vi "Test - Baum Welch algorithm.vi"() -> ()   [LabVIEW 2014, in "HMM.lvlib"]
uses:
  HMM.lvlib
panel:
  out "Estimated HMM 2":T1
  out "#iterations":i32
  out "Probability":dbl[](graph)
  out "Estimated HMM":T1
  out "Observed states":i32[](graph)
  in  "Length of observation":i32
  in  "#iterations":i32=100
  in  "Test HMM":T1
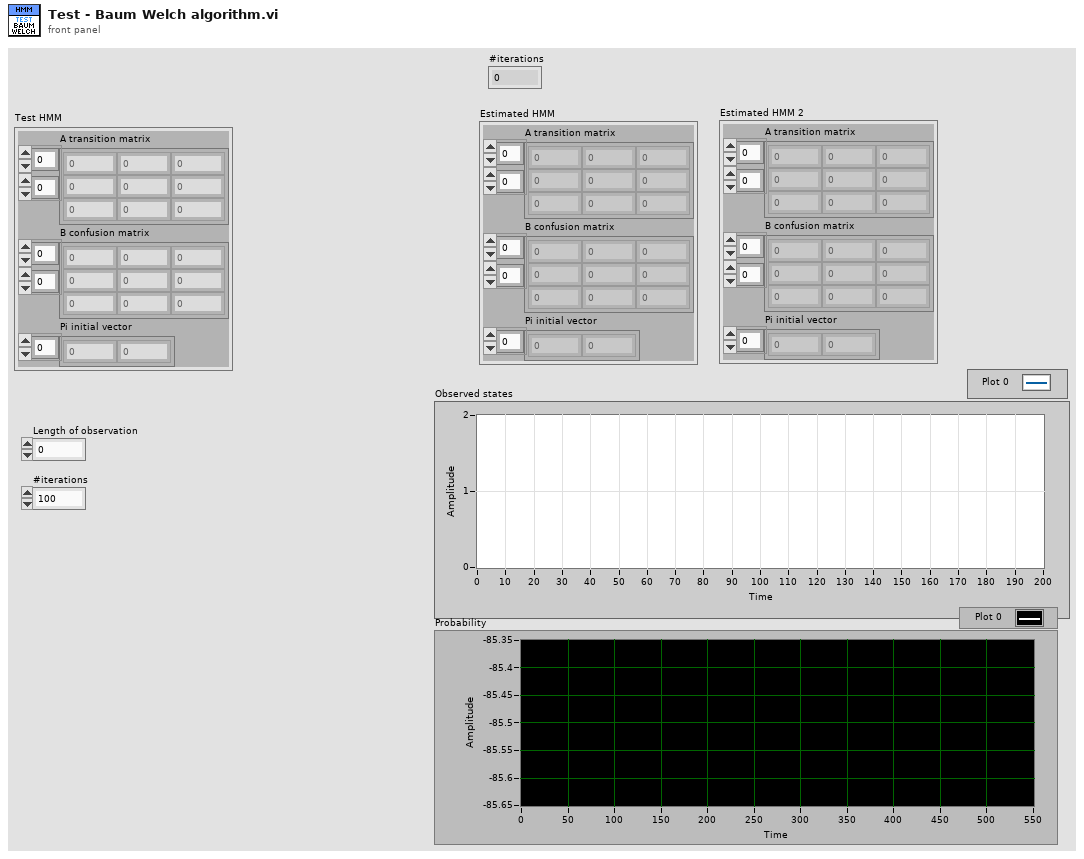
[diagram p1: front panel]
types:
  T1 = cluster{"A transition matrix":dbl[][], "B confusion matrix":dbl[][], "Pi initial vector":dbl[]}
  T2 = typedef "HMM.lvlib/HMM Cluster.ctl" = cluster{"A transition matrix":dbl[][], "B confusion matrix":dbl[][], "Pi initial vector":dbl[]}
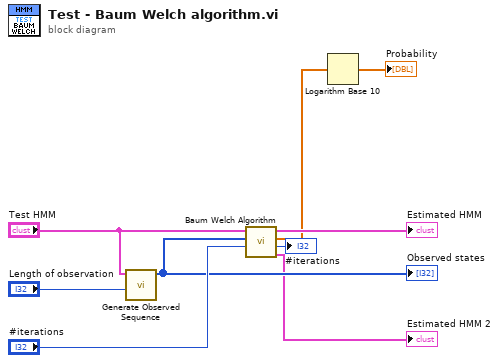
[diagram p0: block diagram]
diagram:
  n1 = call "Generate Observed Sequence.vi"("Length of observation"="Length of observation", "HMM Cluster"="Test HMM") -> ("Observed states"=w5:i32[])  [unwired: 9 in]
  "Observed states" <- w5
  n2 = call "Baum Welch Algorithm.vi"("#iterations"="#iterations", "Observed states"=w5, "Test HMM"="Test HMM") -> ("Pre Estimated HMM"=→"Estimated HMM 2":T2, "#iterations"=→"#iterations":i32, "Probability"=w2:dbl[], "Estimated HMM"=→"Estimated HMM":T2)  [unwired: 5 in]
  n3 = Logarithm Base 10(1:w2) -> (0:→"Probability":dbl[])
